vi "Vechicle Boot Sequence.vi"(0 "Simulate BMS LV":bool=TRUE, 1 "Simulate Motors":bool=TRUE, 2 "Simulate BMS":bool=TRUE, 3 "Simulate Dashboard":bool=TRUE, 4 "Don't irritate me":bool, 5 "Dashboard Control in":T1={"Tractive System"=TRUE, "RTD"=TRUE, "AMS error"=TRUE, "IMD error"=TRUE, "Low Voltage"=0.0, "High Voltage"=0.0} {"High Voltage" scale=0.0..10.0; "Low Voltage" scale=0.0..10.0}, 7 "error in":errorcluster, 10 "CAN Session":T2, 12 "CANOpen Session":refnum<k20>) -> (20 "Left motor Clustered SDO":T4, 21 "Right motor Clustered SDO":T4, 22 "Battery Status":T6, 23 "BMS Low Voltage Status":T3 {"Temp. 0" scale=0.0..80.0; "Temp. 1" scale=0.0..80.0}, 25 "Dashboard Control out":T1={"Tractive System"=TRUE, "RTD"=TRUE, "AMS error"=TRUE, "IMD error"=TRUE, "Low Voltage"=0.0, "High Voltage"=0.0} {"High Voltage" scale=0.0..10.0; "Low Voltage" scale=0.0..10.0}, 27 "error out":errorcluster)   [LabVIEW 2016]
uses:
  RT/Battery Status.ctl
  RT/Clustered SDO.ctl
  RT/BMS Voltage status 2.ctl
  Dashboard Control.ctl
  Program Files (x86)/National Instruments/LabVIEW 2016/examples/robotics/EPOS2 CANOpen Driver/Low Level VIs/Typedefs/CAN Refnum.ctl
  Program Files (x86)/National Instruments/LabVIEW 2016/examples/robotics/EPOS2 CANOpen Driver/Low Level VIs/Typedefs/CAN Session Pointer.ctl
  Program Files (x86)/National Instruments/LabVIEW 2016/examples/robotics/EPOS2 CANOpen Driver/Low Level VIs/Typedefs/CAN Communication References.ctl
  Program Files (x86)/National Instruments/LabVIEW 2016/examples/robotics/EPOS2 CANOpen Driver/Low Level VIs/Typedefs/kill process notifier array.ctl
  Program Files (x86)/National Instruments/LabVIEW 2016/examples/robotics/EPOS2 CANOpen Driver/Low Level VIs/Typedefs/Write Queue.ctl
  Program Files (x86)/National Instruments/LabVIEW 2016/examples/robotics/EPOS2 CANOpen Driver/Low Level VIs/Typedefs/FPGA CAN Frame Cluster.ctl
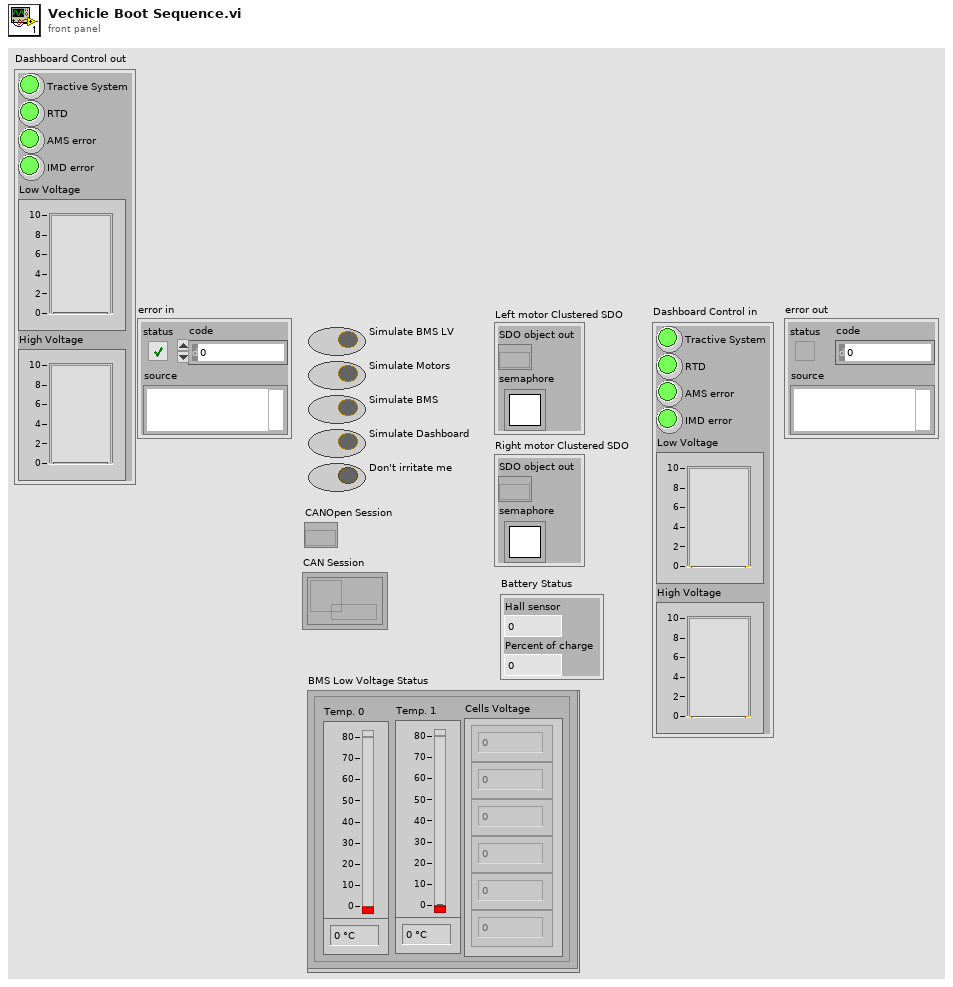
[diagram p1: front panel]
types:
  T1 = typedef "Dashboard Control.ctl" = cluster{"Tractive System":bool, "RTD":bool, "AMS error":bool, "IMD error":bool, "Low Voltage":dbl, "High Voltage":dbl}
  T2 = typedef "CAN Refnum.ctl" = refnum<k1>
  T3 = typedef "BMS Voltage status 2.ctl" = cluster{"Cells Voltage":dbl[], "Temp. 1":u8, "Temp. 0":u8}
  T4 = typedef "Clustered SDO.ctl" = cluster{"SDO object out":refnum<k20>, "semaphore":T5}
  T5 = typedef "Semaphore RefNum" = refnum<k1>
  T6 = typedef "Battery Status.ctl" = cluster{"Hall sensor":i32, "Percent of charge":i16}
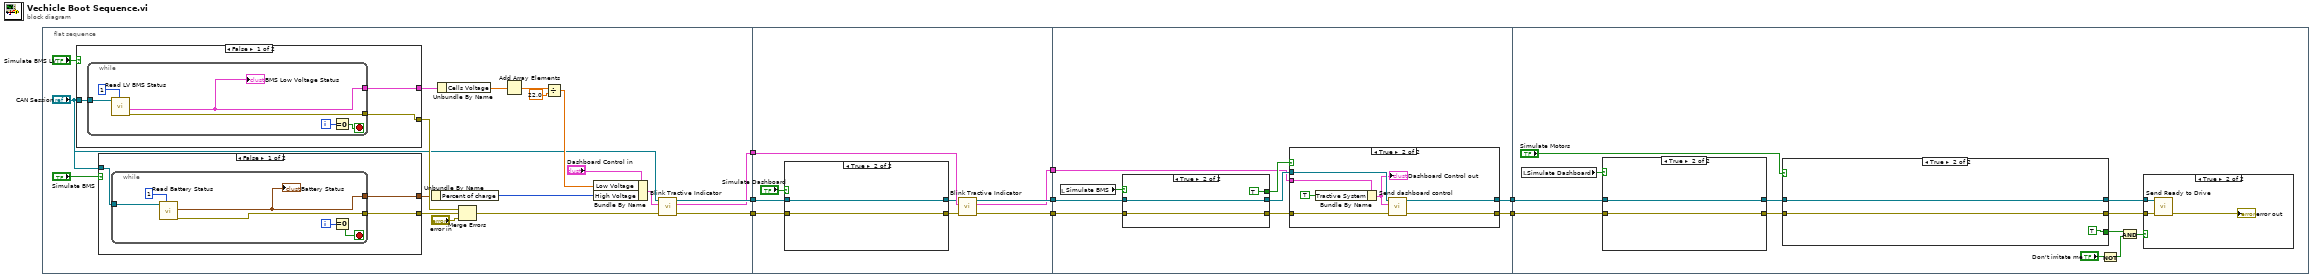
[diagram p0: block diagram]
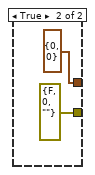
[diagram p2: hidden frame]
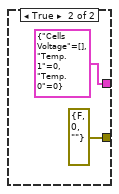
[diagram p3: hidden frame]
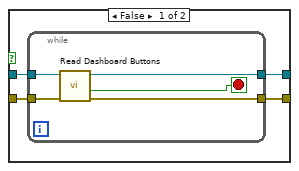
[diagram p4: hidden frame]
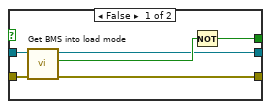
[diagram p6: hidden frame]
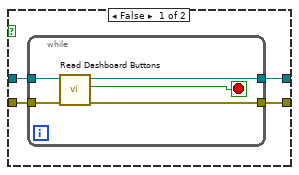
[diagram p7: hidden frame]
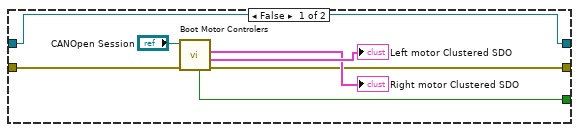
[diagram p9: hidden frame]
diagram:
  n1 = flat-sequence {
    tunnel: [w24] -> w8
    tunnel: [w23] -> w7
    tunnel: [w22] -> w6
    tunnel: w8 -> [w58]
    tunnel: w7 -> [w57]
    tunnel: w6 -> [w55]
    tunnel: [w54] -> w5
    tunnel: [w53] -> w4
    tunnel: [w52] -> w3
    tunnel: w5 -> [w77]
    tunnel: w4 -> [w76]
    tunnel: w3 -> [w72]
    tunnel: [w71] -> w2
    tunnel: [w70] -> w1
    tunnel: w2 -> [w108]
    tunnel: w1 -> [w107]
    frame #0 {
      n2 = case shown="False" "Simulate BMS LV" {
        tunnel: [w41 errorcluster {"status"=FALSE, "code"=0, "source"=""} ("error out")] -> w27
        tunnel: "CAN Session" -> [w40 _]
        tunnel: [w39 T3 {"Cells Voltage"=[], "Temp. 1"=0, "Temp. 0"=0} ("BMS Low Voltage Status")] -> w20
        frame False {
          n3 = while {
            tunnel: [w45] -> w41
            tunnel: w40 -> [w43]
            tunnel: [w44] -> w39
            i -> [w46]
            stop <- w47 stop-if-true
            n4 = call "Read LV BMS Status.vi"("timeout in ms (-1)"=1, "CAN Session In"=w43) -> ("error out"=w45:errorcluster, "BMS Low Voltage Status"=w44:T3)  [unwired: 7 in, 1 out]
            "BMS Low Voltage Status" <- w44
            n5 = Equal To 0?(x=w46) -> (x = 0?=w47:bool)
          }
        }
        frame True {
        }
      }
      n6 = case shown="False" "Simulate BMS" {
        tunnel: [w30 errorcluster {"status"=FALSE, "code"=0, "source"=""} ("error out")] -> w26
        tunnel: "CAN Session" -> [w29 _]
        tunnel: [w28 T6 {"Hall sensor"=0, "Percent of charge"=0} ("Battery Status")] -> w19
        frame False {
          n7 = while {
            tunnel: [w34] -> w30
            tunnel: w29 -> [w33]
            tunnel: [w32] -> w28
            i -> [w35]
            stop <- w36 stop-if-true
            n8 = call "Read Battery Status.vi"("timeout in ms (-1)"=1, "CAN Session In"=w33) -> ("error out"=w34:errorcluster, "Battery Status"=w32:T6)  [unwired: 7 in, 1 out]
            "Battery Status" <- w32
            n9 = Equal To 0?(x=w35) -> (x = 0?=w36:bool)
          }
        }
        frame True {
        }
      }
      n10 = Unbundle By Name(w19) -> ("Percent of charge"=w14:i16)
      n11 = Unbundle By Name(w20) -> ("Cells Voltage"=w18:dbl[])
      n12 = Merge Errors(w27, w26, "error in") -> (w25:errorcluster)
      n13 = Add Array Elements(numeric array=w18) -> (sum=w17:dbl)
      n14 = Divide(x=w17, y=22.0) -> (x/y=w15:dbl)
      n15 = Bundle By Name(cluster="Dashboard Control in", "Low Voltage"=w15, "High Voltage"=w14) -> (w21:T1)
      n16 = call "Blink Tractive Indicator.vi"("error in"=w25, "Dashboard Control in"=w21, "CAN Session In"="CAN Session") -> ("error out"=w24:errorcluster, "Dashboard Control out"=w22:T1, "CAN Session Out"=w23:T2)  [unwired: 6 in]
    }
    frame #1 {
      n17 = case shown="True" "Simulate Dashboard" {
        tunnel: w58 -> [w62 w69]
        tunnel: w57 -> [w61 w68]
        tunnel: [w60 w69] -> w56
        tunnel: [w59 w68] -> w51
        frame False {
          n18 = while {
            tunnel: w62 -> [w67]
            tunnel: w61 -> [w66]
            tunnel: [w65] -> w60
            tunnel: [w63] -> w59
            stop <- w64 stop-if-true
            n19 = call "Read Dashboard Buttons.vi"("error in"=w67, "CAN Session In"=w66) -> ("error out"=w65:errorcluster, "Tractive system activation"=w64:bool, "CAN Session Out"=w63:T2)  [unwired: 6 in, 1 out]
          }
        }
        frame True {
        }
      }
      n20 = call "Blink Tractive Indicator.vi"("error in"=w56, "Dashboard Control in"=w55, "CAN Session In"=w51) -> ("error out"=w53:errorcluster, "Dashboard Control out"=w52:T1, "CAN Session Out"=w54:T2)  [unwired: 6 in]
    }
    frame #2 {
      n21 = local read "Simulate BMS"() -> (w78:bool)
      n22 = case shown="True" w78 {
        tunnel: w76 -> [w93 w96]
        tunnel: [w92 w96] -> w74
        tunnel: w77 -> [w90 w94]
        tunnel: [w89 TRUE] -> w75
        tunnel: [w88 w94] -> w73
        frame False {
          n23 = call "Get BMS into load mode.vi"("error in"=w93, "CAN Session In"=w90) -> ("error out"=w92:errorcluster, "Error"=w91:bool, "CAN Session Out"=w88:T2)  [unwired: 7 in]
          n24 = Not(x=w91) -> (.not. x?=w89:bool)
        }
        frame True {
        }
      }
      n25 = case shown="True" w75 {
        tunnel: w74 -> [w80 w87]
        tunnel: w73 -> [w79 w86]
        tunnel: w72 -> [_ w84]
        tunnel: [w80 w83] -> w71
        tunnel: [w79 w82] -> w70
        frame False {
        }
        frame True {
          n26 = Bundle By Name(cluster=w84, "Tractive System"=TRUE) -> (w81:T1)
          "Dashboard Control out" <- w81
          n27 = call "Send dashboard control.vi"("error in"=w87, "Dashboard Control"=w81, "CAN Session In"=w86) -> ("error out"=w83:errorcluster, "CAN Session Out"=w82:T2)  [unwired: 7 in]
        }
      }
    }
    frame #3 {
      n28 = local read "Simulate Dashboard"() -> (w98:bool)
      n29 = case shown="True" w98 {
        tunnel: w108 -> [w112 w118]
        tunnel: w107 -> [w111 w119]
        tunnel: [w110 w118] -> w106
        tunnel: [w109 w119] -> w100
        frame False {
          n30 = while {
            tunnel: w112 -> [w117]
            tunnel: w111 -> [w116]
            tunnel: [w114] -> w110
            tunnel: [w115] -> w109
            stop <- w113 stop-if-true
            n31 = call "Read Dashboard Buttons.vi"("error in"=w117, "CAN Session In"=w116) -> ("error out"=w114:errorcluster, "Ready to drive"=w113:bool, "CAN Session Out"=w115:T2)  [unwired: 6 in, 1 out]
          }
        }
        frame True {
        }
      }
      n32 = case shown="True" "Simulate Motors" {
        tunnel: [w127 w131] -> w101
        tunnel: [w126 TRUE] -> w102
        tunnel: w106 -> [w125 w131]
        tunnel: w100 -> [w124 w130]
        tunnel: [w124 w130] -> w99
        frame False {
          n33 = call "Boot Motor Controlers.vi"("error in (no error)"=w125, "CANOpen Session in"="CANOpen Session") -> ("error out"=w127:errorcluster, "Left motor Clustered SDO"=→"Left motor Clustered SDO":T4, "Right motor Clustered SDO"=→"Right motor Clustered SDO":T4, "Error"=w126:bool)  [unwired: 5 in, 1 out]
        }
        frame True {
        }
      }
      n34 = Not(x="Don't irritate me") -> (.not. x?=w105:bool)
      n35 = Compound Arithmetic op=AND(w102, w105) -> (w103:bool)
      n36 = case shown="True" w103 {
        tunnel: w99 -> [_ w122]
        tunnel: w101 -> [_ w121]
        frame False {
        }
        frame True {
          n37 = call "Send Ready to Drive.vi"("error in"=w121, "CAN Session In"=w122) -> ("error out"=→"error out":errorcluster)  [unwired: 8 in, 1 out]
        }
      }
    }
  }
